vi "serial.vi"(5 "写入缓冲区":string, 6 "baud rate (9600)":u32=9600 caption="波特率(9600)", 7 "VISA资源名称":refnum<visa-resource-name>) -> (1 "错误输出":errorcluster, 2 "VISA资源名称输出":refnum<visa-resource-name>, 3 "读取缓冲区":string)   [LabVIEW 2023]
uses:
  <vilib>/Instr/_visa.llb/VISA Configure Serial Port (Instr).vi
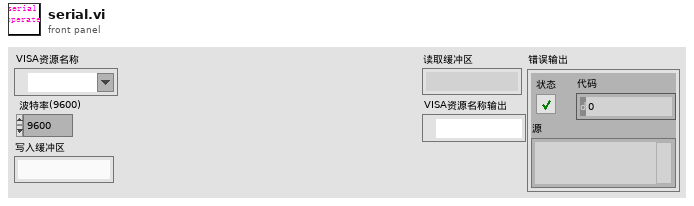
[diagram p1: front panel]
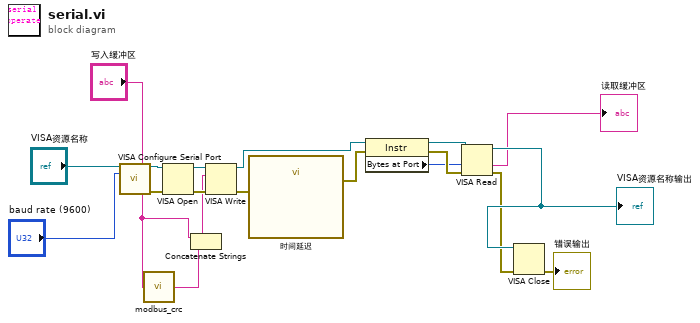
[diagram p0: block diagram]
diagram:
  n1 = call-poly "VISA Configure Serial Port"("VISA resource name"="VISA资源名称", "baud rate (9600)"="baud rate (9600)") -> ("VISA resource name out"=w18:refnum<visa-resource-name>, "error out"=w14:errorcluster)  [unwired: 12 in]
  n2 = call "modbus_crc.vi"("字符串"="写入缓冲区") -> ("十六进制整型字符串"=w3:string)
  n3 = VISA Open(error in (no error)=w14, VISA resource name=w18) -> (VISA resource name=w16:refnum<visa-resource-name>, error out=w13:errorcluster)  [unwired: 3 in]
  n4 = Concatenate Strings("写入缓冲区", w3) -> (w2:string)
  n5 = VISA Write(VISA resource name=w16, write buffer=w2, error in (no error)=w13) -> (VISA resource name out=w15:refnum<visa-resource-name>, error out=w12:errorcluster)  [unwired: 1 out]
  n6 = call "时间延迟"("error in (no error)"=w12) -> ("error out"=w11:errorcluster)  [unwired: 10 in]
  n7 = property class="Instr"(reference=w15, error in=w11) -> (reference out=w10:refnum<visa-resource-name>, error out=w9:errorcluster, "Bytes at Port"=w5:u32)
  n8 = VISA Read(VISA resource name=w10, byte count=w5, error in (no error)=w9) -> (VISA resource name out=w8:refnum<visa-resource-name>, read buffer=→"读取缓冲区":string, error out=w7:errorcluster)  [unwired: 1 out]
  "VISA资源名称输出" <- w8
  n9 = VISA Close(VISA resource name=w8, error in (no error)=w7) -> (error out=→"错误输出":errorcluster)
